vi "fgv_data.vi"() -> ()   [LabVIEW 2017]
uses:
  ctrls/data.ctl
panel:
  in  "data_in":T1 {"steer" scale=0.0..10.0; "speed" scale=0.0..10.0}
  out "data_out":T1 {"steer" scale=0.0..10.0; "speed" scale=0.0..10.0}
  in  "cmd":enum16{"ini", "write", "read"}(ring)
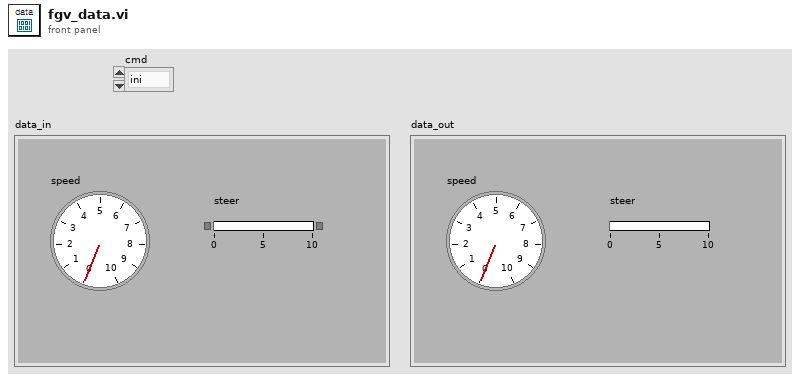
[diagram p1: front panel]
types:
  T1 = typedef "data.ctl" = cluster{"speed":dbl, "steer":dbl}
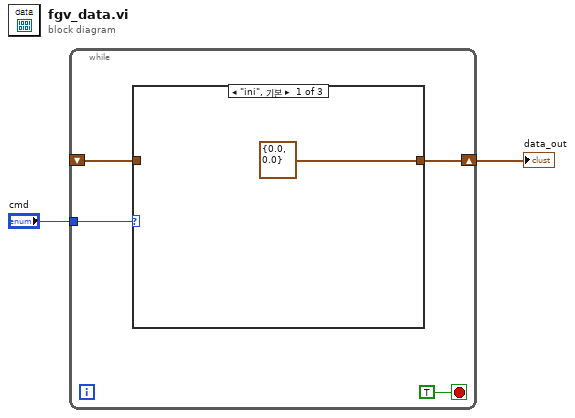
[diagram p0: block diagram]
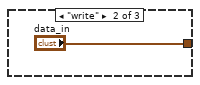
[diagram p2: hidden frame]
diagram:
  n1 = while {
    shift-right: [w4] -> w1
    shift-left: _ -> [w3]
    tunnel: "cmd" -> [w5]
    stop <- TRUE stop-if-true
    n2 = case shown="\"ini\", 기본" w5 {
      tunnel: [T1 {"speed"=0.0, "steer"=0.0} ("data 2") "data_in" w9] -> w4
      tunnel: w3 -> [_ _ w9]
      frame "ini", Default {
      }
      frame "write" {
      }
      frame "read" {
      }
    }
  }
  "data_out" <- w1
